vi "fgv_AOdaqmx.vi"(7 "cmd":T1=enum."init", 8 "error in":errorcluster) -> (0 "error out":errorcluster)   [LabVIEW 2019]
uses:
  _ctrl/init-w-close.ctl
  _ctrl/rw.ctl
  <vilib>/DAQmx/write.llb/DAQmx Write (Analog Wfm 1Chan NSamp).vi
  <vilib>/DAQmx/create/channels.llb/DAQmx Create Channel (AO-Voltage-Basic).vi
  <vilib>/DAQmx/configure/timing.llb/DAQmx Timing (Sample Clock).vi
  <vilib>/DAQmx/miscellaneous.llb/DAQmx Fill In Error Info.vi
panel:
  out "sample mode":i32(ring)=10178 items=["유한 샘플"=10178, "연속 샘플"=10123, "하드웨어 타이밍에 의한 단일 포인트"=12522]
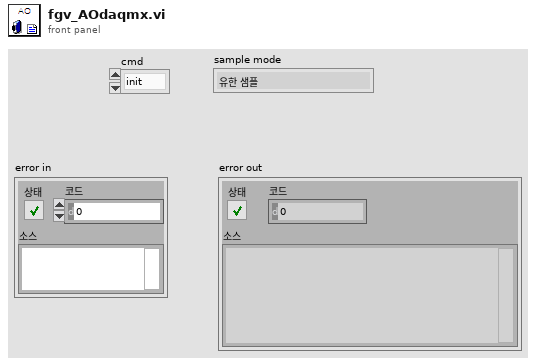
[diagram p1: front panel]
types:
  T1 = typedef "init-w-close.ctl" = enum16{"open", "init", "write", "close"}
  T2 = typedef "rw.ctl" = enum16{"read", "write"}
  T3 = typedef "cDAQ-9269 Config.ctl" = cluster{"Ch":tag, "Max V":dbl, "Min V":dbl, " Rate":dbl, "N pts":i32, "sample mode":i32}
  T4 = typedef "system-status_내구.ctl" = enum16{"Initial", "Update", "Clear"}
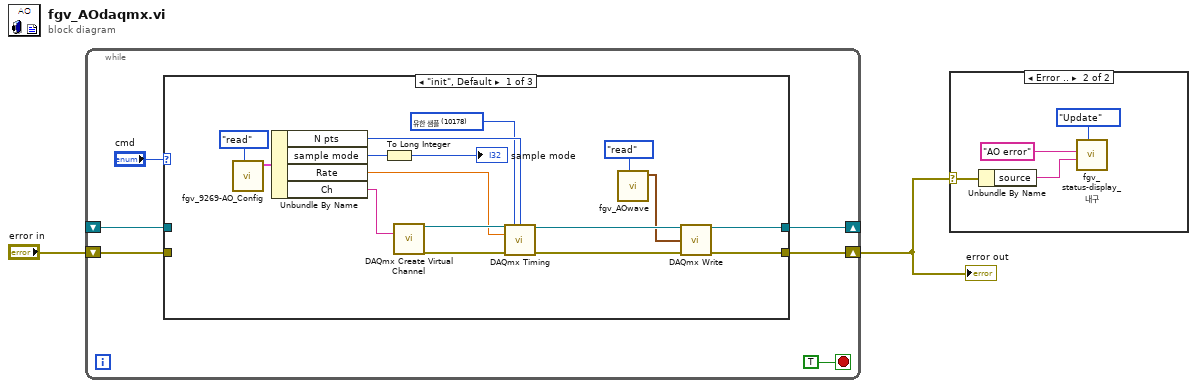
[diagram p0: block diagram]
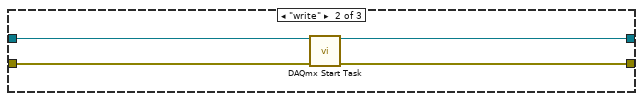
[diagram p3: hidden frame]
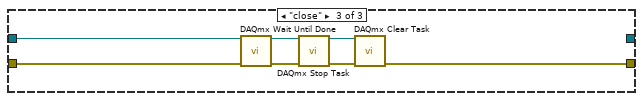
[diagram p4: hidden frame]
diagram:
  n1 = while {
    shift-right: [w6] -> _
    shift-left: _ -> [w3]
    shift-right: [w5] -> w1
    shift-left: "error in" -> [w4]
    stop <- TRUE stop-if-true
    n2 = case shown="\"init\", Default" "cmd" {
      tunnel: [w20 w25 _] -> w6
      tunnel: [w21 w26 w29] -> w5
      tunnel: w4 -> [_ w28 w30]
      tunnel: w3 -> [_ w27 w31]
      frame "init", Default {
        w11 = 10178 items=["유한 샘플"=10178, "연속 샘플"=10123, "하드웨어 타이밍에 의한 단일 포인트"=12522] ("sample mode")
        n3 = call "fgv_9269-AO_Config.vi"("cmd"=rw."read") -> ("config 2"=w12:T3)  [unwired: 9 in, 1 out]
        n4 = Unbundle By Name(w12) -> ("N pts"=w14:i32, "sample mode"=w13:i32, "Rate"=w16:dbl, "Ch"=w17:tag)
        n5 = To Long Integer(number=w13) -> (32bit integer=→"sample mode":i32)
        n6 = call-poly <vilib>:"DAQmx Create Virtual Channel.vi"("physical channels"=w17) -> ("task out"=w23:refnum<k21>, "error out"=w24:errorcluster)  [unwired: 13 in]
        n7 = call-poly <vilib>:"DAQmx Timing.vi"("task/channels in"=w23, "sample mode"=w11, "samples per channel"=w14, "rate"=w16, "error in"=w24) -> ("task out"=w19:refnum<k21>, "error out"=w22:errorcluster)  [unwired: 9 in]
        n8 = call "fgv_AOwave.vi"("cmd"=rw."read") -> ("signal out"=w9:waveform(dbl))  [unwired: 9 in, 1 out]
        n9 = call-poly <vilib>:"DAQmx Write.vi"("task/channels in"=w19, "data"=w9, "error in"=w22) -> ("task out"=w20:refnum<k21>, "error out"=w21:errorcluster)  [unwired: 10 in, 1 out]
      }
      frame "write" {
        n10 = call <vilib>:"DAQmx Start Task.vi"("task/channels in"=w27, "error in"=w28) -> ("task out"=w25:refnum<k21>, "error out"=w26:errorcluster)  [unwired: 12 in]
      }
      frame "close" {
        n11 = call <vilib>:"DAQmx Wait Until Done.vi"("task/channels in"=w31, "error in"=w30) -> ("task out"=w33:refnum<k21>, "error out"=w32:errorcluster)  [unwired: 12 in]
        n12 = call <vilib>:"DAQmx Stop Task.vi"("task/channels in"=w33, "error in"=w32) -> ("task out"=w35:refnum<k21>, "error out"=w34:errorcluster)  [unwired: 12 in]
        n13 = call <vilib>:"DAQmx Clear Task.vi"("task in"=w35, "error in"=w34) -> ("error out"=w29:errorcluster)  [unwired: 13 in]
      }
    }
  }
  "error out" <- w1
  n14 = case shown="Error .." w1 {
    selector: w1 -> [_ w37]
    frame No Error {
    }
    frame Error {
      n15 = Unbundle By Name(w37) -> ("source"=w36:string)
      n16 = call "fgv_status-display_내구.vi"("Mode"=system-status_내구."Update", "detail"=w36, "title"="AO error") -> ()  [unwired: 8 in, 1 out]
    }
  }
